vi "VisionMain.vi"(8 "Y Center":dbl, 9 "X Center":dbl, 10 "Original Plots":T1(array[cluster]), 11 "Plots Captured":T1(array[cluster])) -> (1 "alpha":dbl, 2 "dy":dbl, 3 "dx":dbl)   [LabVIEW 2012]
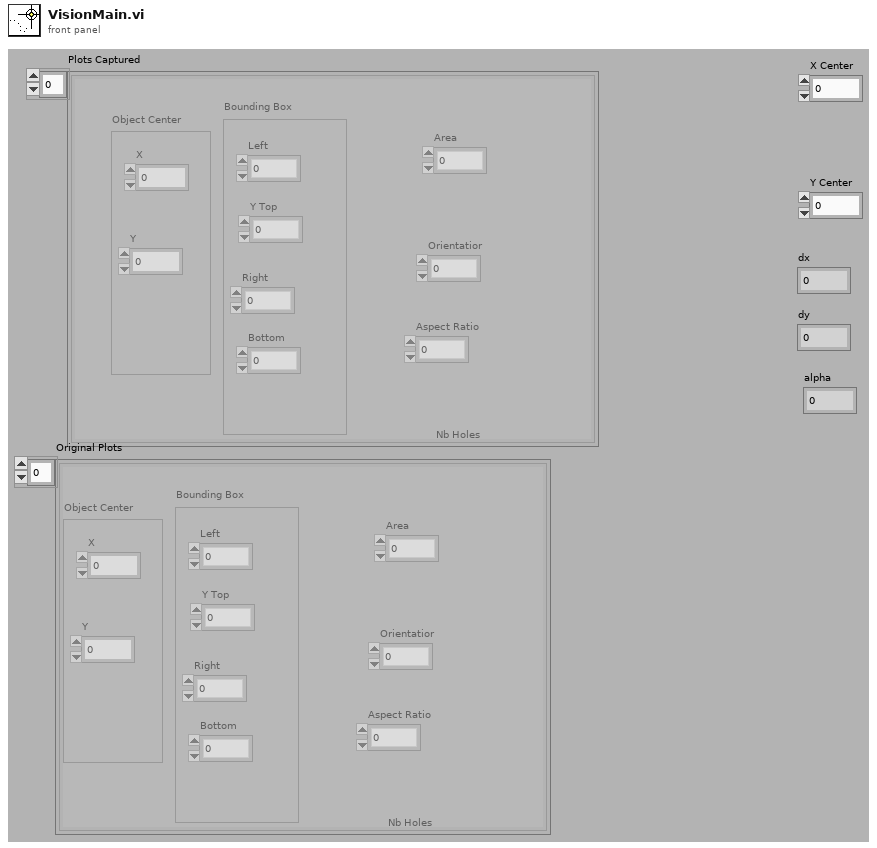
[diagram p1: front panel]
types:
  T1 = cluster{"Object Center":cluster{"X":dbl, "Y":dbl}, "Bounding Box":cluster{"Left":dbl, "Right":dbl, "Bottom":dbl, "Y Top":dbl}, "Area":dbl, "Orientatior":dbl, "Aspect Ratio":dbl, "Nb Holes":dbl}[]
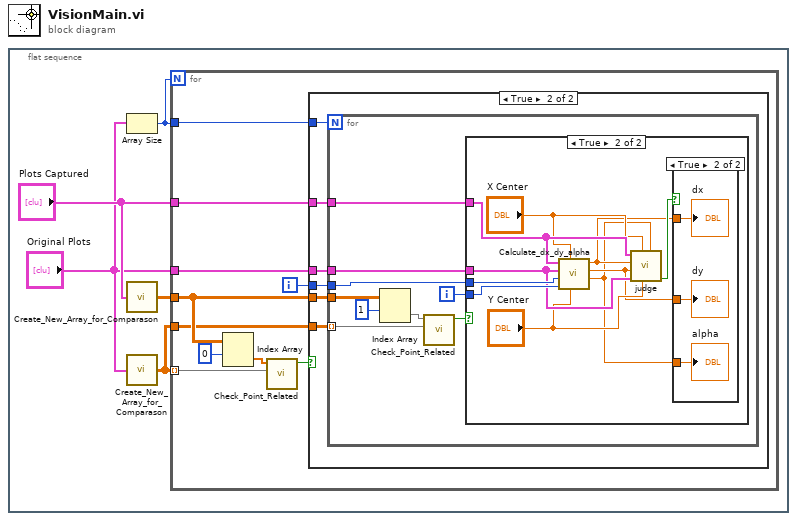
[diagram p0: block diagram]
diagram:
  n1 = flat-sequence {
    frame #0 {
      n2 = Array Size(array="Original Plots") -> (size(s)=w1:i32)
      n3 = call "Create_New_Array_for_Comparason.vi"("Captured Plots"="Plots Captured") -> ("Generated Distance Array"=w5:dbl[][])
      n4 = call "Create_New_Array_for_Comparason.vi"("Captured Plots"="Original Plots") -> ("Generated Distance Array"=w4:dbl[][])
      n5 = for {
        N: w1 -> [_]
        tunnel: w5 -> [w12]
        tunnel: w4 -> [w11] mode=indexing
        tunnel: w4 -> [w10]
        tunnel: "Plots Captured" -> [w9]
        tunnel: "Original Plots" -> [w8]
        tunnel: w1 -> [w6]
        i -> [w7]
        n6 = Index Array(array=w12, index (row)=0) -> (element=w14:dbl[])  [unwired: 1 in]
        n7 = call "Check_Point_Related.vi"("Original Plots"=w11, "Captured Plots"=w14) -> ("result"=w13:bool)  [unwired: 9 in]
        n8 = case shown="True" w13 {
          tunnel: w12 -> [_ w21]
          tunnel: w10 -> [_ w20]
          tunnel: w9 -> [_ w19]
          tunnel: w8 -> [_ w18]
          tunnel: w7 -> [_ w17]
          tunnel: w6 -> [_ w16]
          frame False {
          }
          frame True {
            n9 = for {
              N: w16 -> [_]
              tunnel: w21 -> [w30]
              tunnel: w20 -> [w26] mode=indexing
              tunnel: w19 -> [w25]
              tunnel: w18 -> [w24]
              tunnel: w17 -> [w23]
              i -> [w22]
              n10 = Index Array(array=w30, index (row)=1) -> (element=w28:dbl[])  [unwired: 1 in]
              n11 = call "Check_Point_Related.vi"("Original Plots"=w26, "Captured Plots"=w28) -> ("result"=w27:bool)  [unwired: 9 in]
              n12 = case shown="True" w27 {
                tunnel: w25 -> [_ w38]
                tunnel: w24 -> [_ w37]
                tunnel: w23 -> [_ w40]
                tunnel: w22 -> [_ w39]
                frame False {
                }
                frame True {
                  n13 = call "Calculate_dx_dy_alpha.vi"("c_y"="Y Center", "c_x"="X Center", "Corresponding Point #2"=w39, "Corresponding Point #1"=w40, "Original Plots"=w37, "Captured Plots"=w38) -> ("alpha"=w31:dbl, "dy"=w32:dbl, "dx"=w33:dbl)  [unwired: 3 in]
                  n14 = call "judge.vi"("alpha"=w31, "c_y"="Y Center", "c_x"="X Center", "Original Plots"=w37, "dy"=w32, "dx"=w33, "Captured Plots"=w38) -> ("result"=w34:bool)  [unwired: 4 in]
                  n15 = case shown="True" w34 {
                    tunnel: w33 -> [_ w43]
                    tunnel: w32 -> [_ w42]
                    tunnel: w31 -> [_ w41]
                    frame False {
                    }
                    frame True {
                      "dx" <- w43
                      "dy" <- w42
                      "alpha" <- w41
                    }
                  }
                }
              }
            }
          }
        }
      }
    }
  }
